vi "Search threshold value.vi"(0 "Delta Matrix":T2=[[-1.0, 0.0, 0.0, 0.0, 0.0, 0.0, 0.0, 0.0, 0.0], [0.0, -1.0, 0.0, 0.0, 0.0, 0.0, 0.0, 0.0, 0.0], [0.0, 0.0, 0.0, 0.0, 0.0, 0.0, 0.0, 0.0, 0.0], [0.0, 0.0, 0.0, 0.0, 0.0, 0.0, 0.0, 0.0, 0.0], [10.0, 0.0, 0.0, 0.0, 0.0, 0.0, 0.0, 0.0, 0.0], [10.0, 0.0, 0.0, 0.0, 0.0, 0.0, 0.0, 0.0, 0.0], [0.0, 10.0, 0.0, 0.0, 0.0, 0.0, 0.0, 0.0, 0.0]], 1 "Idx of Mod in Sp IDs":i32[](array[numeric])=[2, 8], 2 "CompID":string[](array[string]), 3 "CompSize":string[](array[string]), 5 "Equations":string[](array[string])=["kd*CI", "kd*GFP", "kd*LacI", "kd*TetR", "(ko__P1*ng__P1*Ko__P1*RNAP)/(1+Ko__P1*RNAP+(Kr__LacI_P1*LacI)^nc__LacI_P1)", "(ko__P2*ng__P2*Ko__P2*RNAP)/(1+Ko__P2*RNAP+(Kr__TetR_P2*TetR)^nc__TetR_P2)", "(ko__Promoter_GFP*ng__Promoter_GFP*Ko__Promoter_GFP*RNAP)/(1+Ko__Promoter_GFP*RNAP+(Kr__CI_Promoter_GFP*CI)^nc__CI_Promoter_GFP)"], 7 "Species Info":string[][](array[string])=[["CI", "", "0"], ["GFP", "", "0"], ["LacI", "", "0"], ["P1", "", "4"], ["P2", "", "2"], ["P3", "", "2"], ["P3_mRNA", "", "0"], ["Promoter_GFP", "", "2"], ["TetR", "", "0"]], 9 "Parameter info":string[][](array[string])=[["ko_r", "Reverse RNAP binding rate", "1", "", "", ""], ["nr", "Initial RNAP count", "30", "", "", ""], ["np", "Stoichiometry of production", "10", "", "", ""], ["kr_r", "Reverse repression binding rate", "1", "", "", ""], ["ka_f", "Forward activation binding rate", "0.0033", "", "", ""], ["kecdiff", "Extracellular diffusion rate", "1", "", "", ""], ["ko", "Open complex production rate", "0.05", "", "", ""], ["kmdiff_f", "Forward membrane diffusion rate", "1", "", "", ""], ["kecd", "Extracellular degradation rate", "0.005", "", "", ""], ["kc_r", "Reverse complex formation rate", "1", "", "", ""], ["kr_f", "Forward repression binding rate", "0.5", "", "", ""], ["ka_r", "Reverse activation binding rate", "1", "", "", ""], ["nc", "Stoichiometry of binding", "2", "", "", ""], ["kao_r", "Reverse activated RNAP binding rate", "1", "", "", ""], ["kd", "Degradation rate", "0.0075", "", "", ""], ["kb", "Basal production rate", "0.0001", "", "", ""], ["ng", "Initial promoter count", "2", "", "", ""], ["ka", "Activated production rate", "0.255", "", "", ""], ["kao_f", "Forward activated RNAP binding rate", "1", "", "", ""], ["kmdiff_r", "Reverse membrane diffusion rate", "0.01", "", "", ""], ["ko_f", "Forward RNAP binding rate", "0.033", "", "", ""], ["kc_f", "Forward complex formation rate", "0.05", "", "", ""], ["High", "", "60", "", "", ""], ["HighTime", "Reverse RNAP binding rate", "2000", "", "", ""], ["HighTime2", "Initial RNAP count", "4000", "", "", ""], ["", "", "", "ko_r", "Reverse RNAP binding rate", "1"], ["", "", "", "nr", "Initial RNAP count", "30"], ["", "", "", "np", "Stoichiometry of production", "10"], ["", "", "", "kr_r", "Reverse repression binding rate", "1"], ["", "", "", "ka_f", "Forward activation binding rate", "0.0033"], ["", "", "", "kecdiff", "Extracellular diffusion rate", "1"], ["", "", "", "ko", "Open complex production rate", "0.05"], ["", "", "", "kmdiff_f", "Forward membrane diffusion rate", "1"], ["", "", "", "kecd", "Extracellular degradation rate", "0.005"], ["", "", "", "kc_r", "Reverse complex formation rate", "1"], ["", "", "", "kr_f", "Forward repression binding rate", "0.5"], ["", "", "", "ka_r", "Reverse activation binding rate", "1"], ["", "", "", "nc", "Stoichiometry of binding", "2"], ["", "", "", "kao_r", "Reverse activated RNAP binding rate", "1"], ["", "", "", "kd", "Degradation rate", "0.0075"], ["", "", "", "kb", "Basal production rate", "0.0001"], ["", "", "", "ng", "Initial promoter count", "2"], ["", "", "", "ka", "Activated production rate", "0.255"], ["", "", "", "kao_f", "Forward activated RNAP binding rate", "1"], ["", "", "", "kmdiff_r", "Reverse membrane diffusion rate", "0.01"], ["", "", "", "ko_f", "Forward RNAP binding rate", "0.033"], ["", "", "", "kc_f", "Forward complex formation rate", "0.05"], ["", "", "", "High", "", "60"], ["", "", "", "HighTime", "Reverse RNAP binding rate", "2000"], ["", "", "", "HighTime2", "Initial RNAP count", "4000"]], 11 "Local Parameter Info":string[][](array[string])=[["kd", "0.0075", "0.0075", "0.0075"], ["kd", "0.0075", "0.0075", "0.0075"], ["kd", "0.0075", "0.0075", "0.0075"], ["kd", "0.0075", "0.0075", "0.0075"], ["RNAP", "30", "0.0075", "0.0075"], ["ng__P1", "4", "0.0075", "0.0075"], ["Ko__P1", "0.033", "0.0075", "0.0075"], ["ko__P1", "0.05", "0.0075", "0.0075"], ["nc__LacI_P1", "2", "0.0075", "0.0075"], ["Kr__LacI_P1", "0.5", "0.0075", "0.0075"], ["RNAP", "30", "0.0075", "0.0075"], ["ng__P2", "2", "0.0075", "0.0075"], ["Ko__P2", "0.033", "0.0075", "0.0075"], ["ko__P2", "0.05", "0.0075", "0.0075"], ["nc__TetR_P2", "2", "0.0075", "0.0075"], ["Kr__TetR_P2", "0.5", "0.0075", "0.0075"], ["RNAP", "30", "0.0075", "0.0075"], ["ng__Promoter_GFP", "2", "0.0075", "0.0075"], ["Ko__Promoter_GFP", "0.033", "0.0075", "0.0075"], ["ko__Promoter_GFP", "0.05", "0.0075", "0.0075"], ["nc__CI_Promoter_GFP", "2", "0.0075", "0.0075"], ["Kr__CI_Promoter_GFP", "0.5", "0.0075", "0.0075"], ["0.0075", "0.0075", "kd", "0.0075"], ["0.0075", "0.0075", "kd", "0.0075"], ["0.0075", "0.0075", "kd", "0.0075"], ["0.0075", "0.0075", "kd", "0.0075"], ["0.0075", "0.0075", "RNAP", "30"], ["0.0075", "0.0075", "ng__P1", "4"], ["0.0075", "0.0075", "Ko__P1", "0.033"], ["0.0075", "0.0075", "ko__P1", "0.05"], ["0.0075", "0.0075", "nc__LacI_P1", "2"], ["0.0075", "0.0075", "Kr__LacI_P1", "0.5"], ["0.0075", "0.0075", "RNAP", "30"], ["0.0075", "0.0075", "ng__P2", "2"], ["0.0075", "0.0075", "Ko__P2", "0.033"], ["0.0075", "0.0075", "ko__P2", "0.05"], ["0.0075", "0.0075", "nc__TetR_P2", "2"], ["0.0075", "0.0075", "Kr__TetR_P2", "0.5"], ["0.0075", "0.0075", "RNAP", "30"], ["0.0075", "0.0075", "ng__Promoter_GFP", "2"], ["0.0075", "0.0075", "Ko__Promoter_GFP", "0.033"], ["0.0075", "0.0075", "ko__Promoter_GFP", "0.05"], ["0.0075", "0.0075", "nc__CI_Promoter_GFP", "2"], ["0.0075", "0.0075", "Kr__CI_Promoter_GFP", "0.5"]], 12 "Inputs":T1={"Start at"=0.0, "Increment of"=5.0, "Stop at"=15.0, "No. of iterations"=10.0, "Assumed Time Delay"=800.0, "Th high"=0.0, "Verification RT"=1000.0, "Settling Time"=10, "Name of Output"="GFP", "Th Low"=90.0}, 13 "ModTimeSym":string) -> (4 "Estimated T-delay":i32, 6 "Th-High":dbl, 8 "ET-Delay-SD":dbl format="%0.2f", 10 "E-OC-Th-High":dbl format="%#_4g", 14 "E-OC-Th-Low":dbl, 15 "Th-Low":dbl)   [LabVIEW 2014]
doc: "This VI checks for the possible threshold value for two input genetic circuits. If any possible threshold value is detected, it triggers \"Verify threshold value by repeated iteration.vi\" to perform iterations and verify the level of consistency. \n\n\nLimitations:\n* Index of output protein is hard coded to GFP\n* Input combinations are hard coded for two input circuits\n*\n\nNote: \nLimitations:\n* Index of output protein is hard coded to GFP.\n* Input combinations are hard coded for two input circuits.\n\nDesigned by HB\nhaba@dtu.dk"
uses:
  <vilib>/Analysis/Matrix/Datatypes/RealMatrix.ctl
  Threshold Set.ctl
  ValSubsCtrl.ctl
  VerifyThreshInpCtrl.ctl
  Trigger Status Bar.vi
  <vilib>/Analysis/Matrix/Numeric/Conversions/Matrix To Array - RM.vi
  <vilib>/gmath/NI_Gmath.lvlib
  <vilib>/Analysis/Matrix/NI_Matrix.lvlib
panel:
  out "TIME IN MS":i32
  out "UD-OC-Th-Low":dbl
  out "OP Cons-Int":dbl
  in  "ThLow":bool
  out "Verification RT":dbl=1000.0
  out "Combinations":string[](array[string])
  out "UD-OC-Th-High":dbl
  out "output variable":u8
  out "Comb":string
  out "Init Sp State":i32[](array[numeric])
  out "Pos Thresh":dbl
  out "O/p cross":bool
  out "C-o/p":dbl
  out "Nxt Level":dbl
  out "Init OP Conc":dbl
  out "OP Data":dbl[](array[numeric])
  out "idx of OP":i32
  out "Level Run":i32
  out "Time Delay":dbl
  out "Levels":dbl format="%#_2g"
  out "Stop at":dbl
  out "Increment of":dbl
  out "Runs":dbl
  out "Start at":dbl
  out "Mod data":dbl[](array[numeric])
  out "Log Data matrix":dbl[][](array[numeric]) format="%0.3f"
  out "Sp Ids":string[](array[string])=["CI", "GFP", "LacI", "P1", "P2", "P3", "P3_mRNA", "Promoter_GFP", "TetR"]
  out "All Param Names":string[](array[string])
  out "All Param Values":string[](array[string])
  out "Nxt Sp State (N)":i32[](array[numeric])
  out "Nxt Sp State (S)":string[](array[string])
  out "Nxt T":dbl
  out "Sum of Propensities for U":dbl
  out "Reac to execute":dbl[](array[numeric])
  out "Output Equations":string[](array[string])
  out "Log Data":dbl[](array[numeric])
  out "Sum>a0*r2":bool
  out "Reac IDx":i32
  out "a0*r2":dbl
  out "r1":dbl
  out "a0":dbl
  out "Propensities":dbl[](array[numeric])
  out "L_cnt":i32
  out "T":dbl[](array[numeric])
  out "tau":dbl
  out "r2":dbl
  # "Inputs to \"iterative average calc July 20\"vi"
  # "Outputs from \"iterative average calc July 20\"vi"
  # "Delta Matrix"
  # "Start at"
  # "T-Delay"
  # "OP Consistency"
  # "Pos Thresh"
  # "Idx of Mod in Sp IDs"
  # "Runs"
  # "idx of OP"
  # "init Sp State"
  # "Equations"
  # "All Param Names"
  # "All Param Values"
  # "Sp IDs"
  # "Init OP Conc"
  # "Input concentration values"
  # "% Acceptance of consistency"
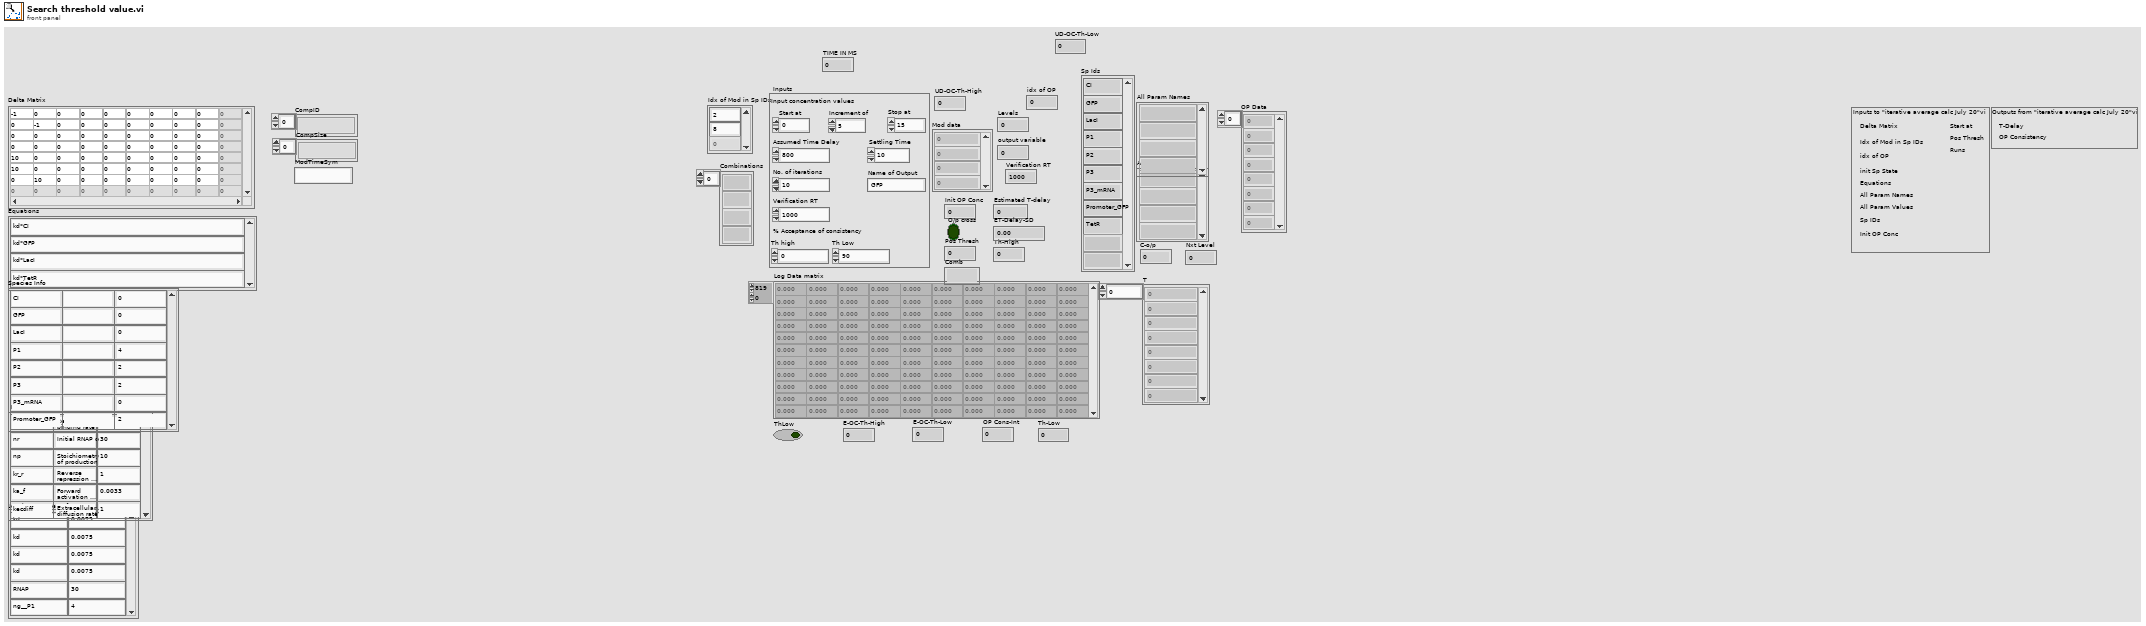
[diagram p1: front panel]
types:
  T1 = typedef "Threshold Set.ctl" = cluster{"Start at":dbl, "Increment of":dbl, "Stop at":dbl, "No. of iterations":dbl, "Assumed Time Delay":dbl, "Th high":dbl, "Verification RT":dbl, "Settling Time":i32, "Name of Output":string, "Th Low":dbl}
  T2 = typedef "NI_Matrix.lvlib/RealMatrix.ctl" = dbl[][]
  T3 = typedef "ValSubsCtrl.ctl" = cluster{"All Param Names":string[], "All Param Values":string[], "Sp IDs":string[], "Sp States":string[], "Input Equations":string[], "CompID":string[], "CompSize":string[], "T-Sym":string, "T":dbl}
  T4 = typedef "VerifyThreshInpCtrl.ctl" = cluster{"Delta Matrix ":T2, "Idx of Mod in Sp IDs ":i32[], "idx of OP ":i32, "Init Sp State ":i32[], "Equations ":string[], "All Param Names ":string[], "All Param Values ":string[], "Sp Ids ":string[], "Start at ":dbl, "Pos Thresh ":dbl, "Runs ":dbl, "Init OP Conc ":dbl, "Comb ":string, "Verification RT ":dbl, "CompID":string[], "CompSize":string[], "ModTimeSym":string, "Settling Time":i32}
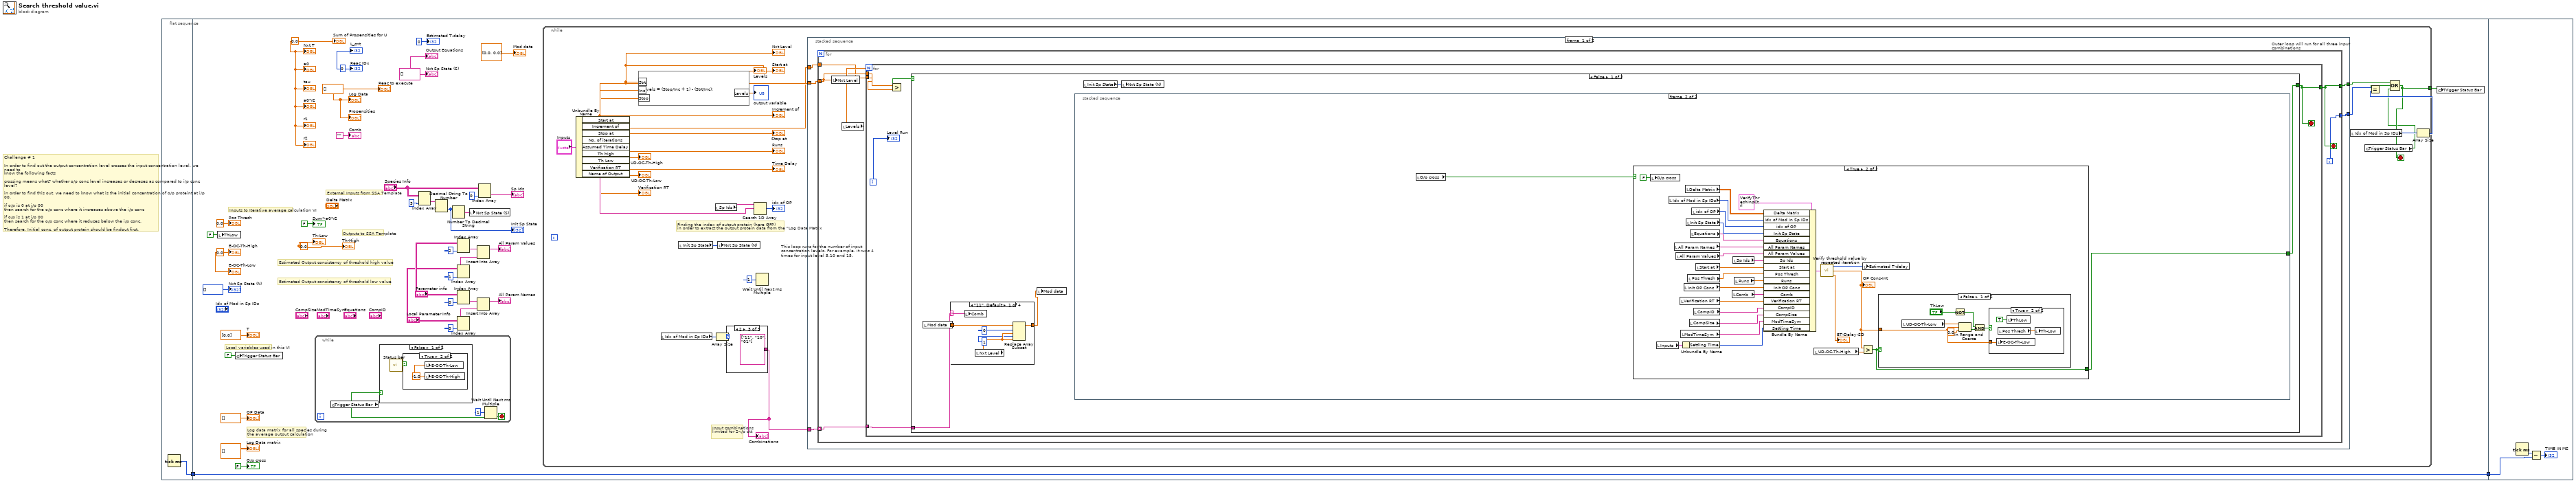
[diagram p0: block diagram]
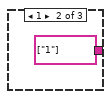
[diagram p5: hidden frame]
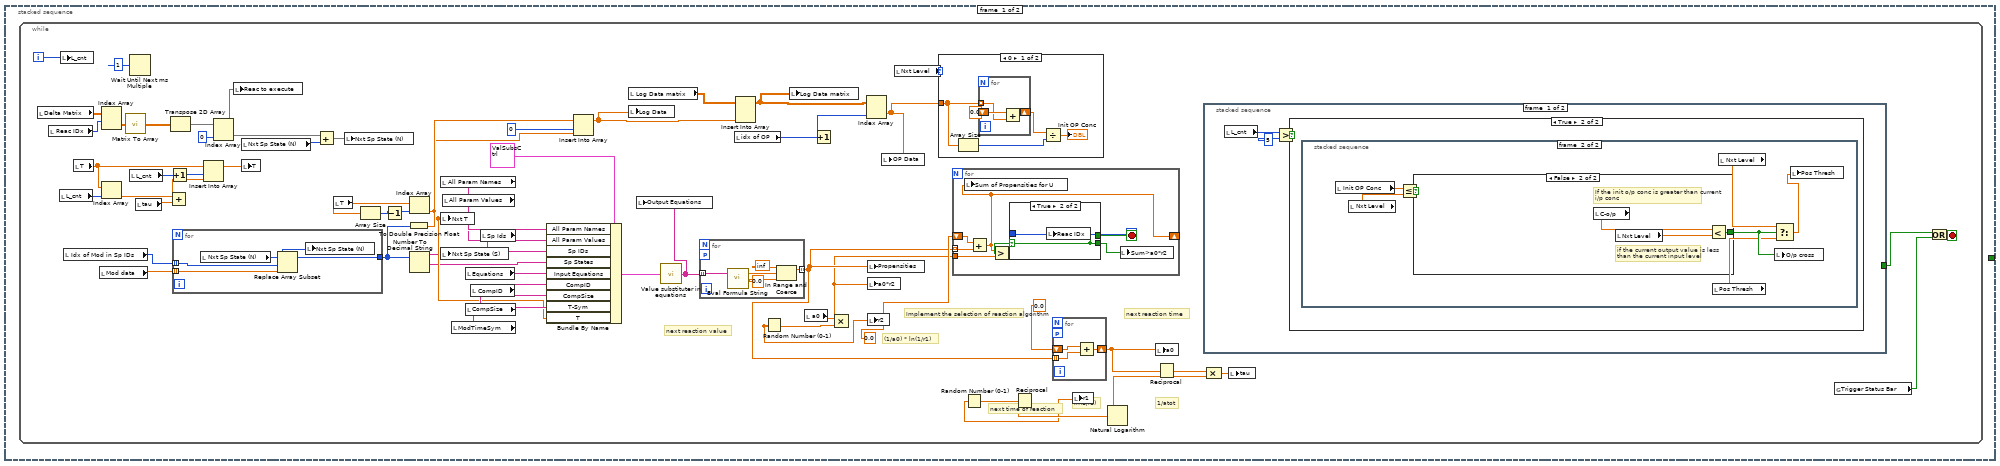
[diagram p6: hidden frame]
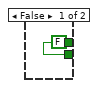
[diagram p8: hidden frame]
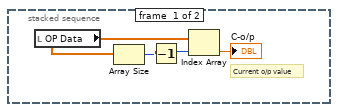
[diagram p10: hidden frame]
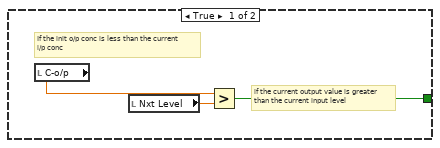
[diagram p11: hidden frame]
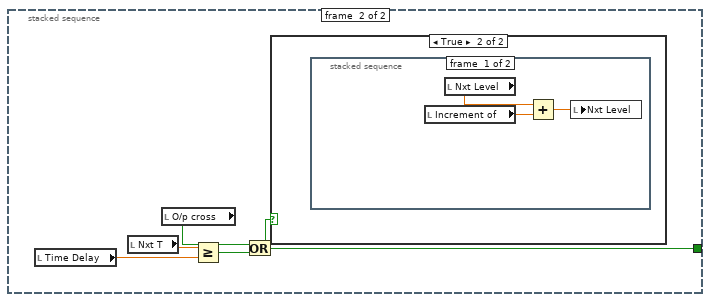
[diagram p12: hidden frame]
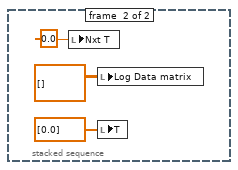
[diagram p14: hidden frame]
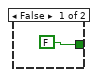
[diagram p15: hidden frame]
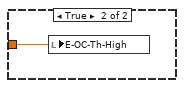
[diagram p17: hidden frame]
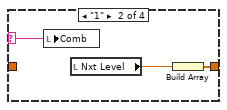
[diagram p18: hidden frame]
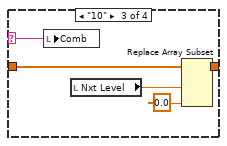
[diagram p19: hidden frame]
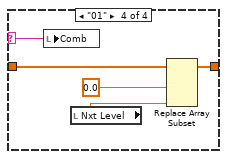
[diagram p20: hidden frame]
diagram:
  # "Challenge # 1\n\nIn order to find out the output concentration level crosses the input concentration level, we need to \nknow the following facts\n\ncrossing means what? whether o/p conc level increases or decreses as compared to i/p conc level?\n\nin order to find this out, we need to know what is the initial concentration of o/p proteint at i/p 00.\n\nif o/p is 0 at i/p 00\nthen search for the o/p conc where it increases above the i/p conc\n\nif o/p is 1 at i/p 00\nthen search for the o/p conc where it reduces below the i/p conc.\n\nTherefore, Initial conc. of output protein should be findout first."
  n1 = flat-sequence {
    tunnel: [w3] -> w1
    tunnel: [w4] -> w2
    tunnel: w1 -> [w4]
    tunnel: w2 -> [w281]
    frame #0 {
      n2 = Tick Count (ms)() -> (millisecond timer value=w3:u32)
    }
    frame #1 {
      w6 = 0.0 ("OP Consistency (%)")
      w5 = 0.0 ("Threshold Value")
      w17 = dbl[] [] ("Reac to execute")
      w28 = 0.0 ("a0")
      w29 = 0 ("L_cnt")
      w30 = string[] [] ("Nxt Sp State (S)")
      # "Estimated Output consistency of threshold low value"
      # "Estimated Output consistency of threshold high value"
      # "Local variables used in this VI"
      # "Outputs to SSA Template"
      # "Log data matrix for all species during \nthe average output calculation"
      # "Inputs to Iterative average calculation VI"
      # "External Inputs from SSA Template"
      n3 = local write "ThLow"(FALSE ("ThLow")) -> ()
      n4 = global write "Trigger Status Bar.vi" "Trigger Status Bar"(FALSE ("Trigger Status Bar")) -> ()
      n5 = while {
        stop <- w44 stop-if-true
        n6 = global read "Trigger Status Bar.vi" "Trigger Status Bar"() -> (w44:bool)
        n7 = case shown="False" w44 {
          frame False {
            n8 = call "Status bar.vi"() -> ("Cancel Button 2"=w45:bool)  [unwired: 11 in]
            n9 = case shown="True" w45 {
              frame False {
              }
              frame True {
                w46 = -1.0 ("OP Consistency (%)")
                n10 = local write "E-OC-Th-Low"(w46) -> ()
                n11 = local write "E-OC-Th-High"(w46) -> ()
              }
            }
          }
          frame True {
          }
        }
        n12 = Wait Until Next ms Multiple(millisecond multiple=u32 1) -> ()  [unwired: 1 out]
      }
      n13 = Index Array(array="Species Info", index (col)=3 ("disabled index (col)")) -> (element=w24:string[])  [unwired: 1 in]
      n14 = Decimal String To Number(string=w24) -> (number=w21:i32[])  [unwired: 2 in, 1 out]
      "Init Sp State" <- w21
      n15 = Number To Decimal String(number=w21) -> (decimal integer string=w20:string[])  [unwired: 1 in]
      n16 = Index Array(array="Parameter info", index (col)=2 ("disabled index (col)")) -> (element=w36:string[])  [unwired: 1 in]
      n17 = Index Array(array="Local Parameter Info", index (col)=1 ("disabled index (col)")) -> (element=w35:string[])  [unwired: 1 in]
      n18 = Index Array(array="Parameter info", index (col)=0 ("disabled index (col)")) -> (element=w38:string[])  [unwired: 1 in]
      n19 = Index Array(array="Local Parameter Info", index (col)=0 ("disabled index (col)")) -> (element=w37:string[])  [unwired: 1 in]
      n20 = local write "Nxt Sp State (S)"(w20) -> ()
      n21 = Insert Into Array(array=w36, new element=w35) -> (→"All Param Values":string[])  [unwired: 1 in]
      n22 = Insert Into Array(array=w38, new element=w37) -> (→"All Param Names":string[])  [unwired: 1 in]
      n23 = Index Array(array="Species Info", index (col)=0 ("disabled index (col)")) -> (element=→"Sp Ids":string[])  [unwired: 1 in]
      n24 = while {
        tunnel: [w65] -> w8
        stop <- w65 stop-if-true
        # "Input combinations\nlimited for 2-i/p ckt"
        # "Finding the index of output protein (here GFP)\nin order to extract the output protein data from the \"Log Data Matrix"
        n25 = Unbundle By Name("Inputs") -> ("Start at"=w49:dbl, "Increment of"=w52:dbl, "Stop at"=w47:dbl, "No. of iterations"=→"Runs":dbl, "Assumed Time Delay"=→"Time Delay":dbl, "Th high"=→"UD-OC-Th-High":dbl, "Th Low"=→"UD-OC-Th-Low":dbl, "Verification RT"=→"Verification RT":dbl, "Name of Output"=w59:string)
        "Start at" <- w49
        "Increment of" <- w52
        "Stop at" <- w47
        "Nxt Level" <- w49
        n26 = formula code="Levels = (Stop/Inc + 1) - (Strt/Inc);"("Strt"=w49, "Inc"=w52, "Stop"=w47) -> ("Levels"=→"Levels" →"output variable":dbl)
        n27 = local read "Idx of Mod in Sp IDs"() -> (w62:i32[])
        n28 = local read "Init Sp State"() -> (w61:i32[])
        n29 = local read "Sp Ids"() -> (w57:string[])
        n30 = Array Size(array=w62) -> (size(s)=w63:i32)
        n31 = local write "Nxt Sp State (N)"(w61) -> ()
        n32 = case shown="2" w63 {
          tunnel: [_ string[] ["1"] string[] ["11", "10", "01"]] -> w48
          frame 0, Default {
          }
          frame 1 {
          }
          frame 2 {
          }
        }
        "Combinations" <- w48
        n33 = Search 1D Array(1D array=w57, element=w59) -> (index of element=→"idx of OP":i32)  [unwired: 1 in]
        n34 = Wait Until Next ms Multiple(millisecond multiple=u32 1) -> ()  [unwired: 1 out]
        n35 = stacked-sequence {
          tunnel: [w78 _] -> w70
          tunnel: [w77 _] -> w71
          tunnel: w49 -> [w76 _]
          tunnel: w48 -> [w75 _]
          tunnel: w47 -> [w74 _]
          frame #0 {
            n36 = for "Outer loop will run for all three input combinations" {
              tunnel: w75 -> [w84] mode=indexing
              tunnel: w76 -> [w80]
              tunnel: [w82] -> w78
              tunnel: [w81] -> w77
              tunnel: w74 -> [w79]
              i -> [w81]
              stop <- w82 stop-if-true
              n37 = local write "Nxt Level"(w80) -> ()
              n38 = local read "Levels"() -> (w83:dbl)
              n39 = for "This loop runs for the number of input concentration levels. For example, it runs 4 times for input level 5,10 and 15." {
                N: w83 -> [_]
                tunnel: w84 -> [w90]
                tunnel: [w87] -> w82
                tunnel: w80 -> [w86]
                tunnel: w79 -> [w85]
                i -> [w89]
                stop <- w87 stop-if-true
                n40 = Greater?(x=w86, y=w85) -> (0:w88:bool)
                n41 = case shown="False" w88 {
                  selector: w88 -> [_ w279]
                  tunnel: w90 -> [w95 _]
                  tunnel: [w94 w279] -> w87
                  frame False {
                    n42 = local read "Mod data"() -> (w92:dbl[])
                    n43 = case shown="\"11\", Default" w95 {
                      selector: w95 -> [w260 w266 w269 w274]
                      tunnel: w92 -> [w265 _ w273 w278]
                      tunnel: [w264 w267 w272 w277] -> w93
                      frame "11", Default {
                        n44 = local write "Comb"(w260) -> ()
                        n45 = local read "Nxt Level"() -> (w263:dbl)
                        n46 = Replace Array Subset(array=w265, new element #1=w263, index #1=0 ("index"), new element #2=w263, index #2=1 ("index")) -> (w264:dbl[])
                      }
                      frame "1" {
                        n47 = local write "Comb"(w266) -> ()
                        n48 = local read "Nxt Level"() -> (w268:dbl)
                        n49 = Build Array(w268) -> (w267:dbl[])
                      }
                      frame "10" {
                        n50 = local write "Comb"(w269) -> ()
                        n51 = local read "Nxt Level"() -> (w270:dbl)
                        n52 = Replace Array Subset(array=w273, new element #1=w270, new element #2=0.0 ("new element/subarray")) -> (w272:dbl[])  [unwired: 2 in]
                      }
                      frame "01" {
                        n53 = local write "Comb"(w274) -> ()
                        n54 = local read "Nxt Level"() -> (w275:dbl)
                        n55 = Replace Array Subset(array=w278, new element #1=0.0 ("new element/subarray"), new element #2=w275) -> (w277:dbl[])  [unwired: 2 in]
                      }
                    }
                    n56 = local write "Mod data"(w93) -> ()
                    n57 = stacked-sequence {
                      tunnel: [_ w219] -> w94
                      frame #0 {
                        n58 = while {
                          i -> [w156]
                          stop <- w153 stop-if-true
                          # "Implement the selection of reaction algorithm"
                          # "(1/a0) * ln(1/r1)"
                          # "1/atot"
                          # "ln(1/r1)"
                          # "next reaction time"
                          # "next time of reaction"
                          # "next reaction value"
                          n59 = local read "Delta Matrix"() -> (w109:T2)
                          n60 = local read "Reac IDx"() -> (w108:i32)
                          n61 = local read "L_cnt"() -> (w124:i32)
                          n62 = local write "L_cnt"(w156) -> ()
                          n63 = local read "Idx of Mod in Sp IDs"() -> (w150:i32[])
                          n64 = local read "T"() -> (w113:dbl[])
                          n65 = local read "Mod data"() -> (w151:dbl[])
                          n66 = Index Array(array=w109, index (row)=w108) -> (element=w107:T2)  [unwired: 1 in]
                          n67 = Index Array(array=w113, index=w124) -> (element=w122:dbl)
                          n68 = call-poly <vilib>:"Matrix To Array.vi"("Real Matrix"=w107) -> ("Real 2D Array"=w106:dbl[][])
                          n69 = local read "L_cnt"() -> (w120:i32)
                          n70 = Wait Until Next ms Multiple(millisecond multiple=u32 1) -> ()  [unwired: 1 out]
                          n71 = local read "tau"() -> (w123:dbl)
                          n72 = Add(x=w122, y=w123) -> (x+y=w119:dbl)
                          n73 = Increment(x=w120) -> (x+1=w121:i32)
                          n74 = Transpose 2D Array(2D array=w106) -> (transposed array=w105:dbl[][])
                          n75 = for {
                            tunnel: w150 -> [w186] mode=indexing
                            tunnel: w151 -> [w185] mode=indexing
                            tunnel: [w184] -> w143
                            n76 = local read "Nxt Sp State (N)"() -> (w187:i32[])
                            n77 = Replace Array Subset(array=w187, new element=w185, index=w186) -> (w184:i32[])
                            n78 = local write "Nxt Sp State (N)"(w184) -> ()
                          }
                          n79 = Insert Into Array(array=w113, index=w121, new element=w119) -> (w118:dbl[])
                          n80 = Index Array(array=w105, index (col)=0 ("disabled index (col)")) -> (element=w101:dbl[])  [unwired: 1 in]
                          n81 = local write "Reac to execute"(w101) -> ()
                          n82 = local read "Nxt Sp State (N)"() -> (w103:i32[])
                          n83 = local write "T"(w118) -> ()
                          n84 = Add(x=w101, y=w103) -> (x+y=w102:dbl[])
                          n85 = local read "T"() -> (w149:dbl[])
                          n86 = local write "Nxt Sp State (N)"(w102) -> ()
                          n87 = Array Size(array=w149) -> (size(s)=w148:i32)
                          n88 = Decrement(x=w148) -> (x-1=w147:i32)
                          n89 = Index Array(array=w149, index=w147) -> (element=w130:dbl)
                          n90 = To Double Precision Float(number=w143) -> (double precision float=w145:dbl[])
                          n91 = Number To Decimal String(number=w143) -> (decimal integer string=w129:string[])  [unwired: 1 in]
                          n92 = local read "All Param Names"() -> (w137:string[])
                          n93 = local write "Nxt T"(w130) -> ()
                          n94 = local write "Nxt Sp State (S)"(w129) -> ()
                          n95 = local read "All Param Values"() -> (w136:string[])
                          n96 = local read "ModTimeSym"() -> (w141:string)
                          n97 = local read "Equations"() -> (w138:string[])
                          n98 = local read "CompSize"() -> (w140:string[])
                          n99 = local read "CompID"() -> (w139:string[])
                          n100 = local read "Sp Ids"() -> (w135:string[])
                          n101 = Bundle By Name(cluster=T3 {"All Param Names"=["k1"], "All Param Values"=["1.5"], "Sp IDs"=["S1", "S2", "S3"], "Sp States"=["0.000000", "0.000000", "0.000000"], "Input Equations"=["C*k1*S1", "1.5*exp(time)^(-1)"], "CompID"=["C"], "CompSize"=["3.0"], "T-Sym"="time", "T"=0.0} ("Cluster"), "All Param Names"=w137, "All Param Values"=w136, "Sp IDs"=w135, "Sp States"=w129, "Input Equations"=w138, "CompID"=w139, "CompSize"=w140, "T-Sym"=w141, "T"=w130) -> (w134:T3)
                          n102 = Insert Into Array(array=w145, index=0, new element=w130) -> (w142:dbl[])
                          n103 = local read "Log Data matrix"() -> (w144:dbl[][])
                          n104 = local write "Log Data"(w142) -> ()
                          n105 = call "Value substituter in equations.vi"("Cluster"=w134) -> ("Output Equations"=w131:string[])
                          n106 = local write "Output Equations"(w131) -> ()
                          n107 = for {
                            tunnel: w131 -> [w183] mode=indexing
                            tunnel: [w179] -> w111 mode=indexing
                            workers-P: _ -> [_]
                            n108 = call <vilib>:"Eval Formula String.vi"("formula"=w183) -> ("y value"=w180:dbl)  [unwired: 1 in, 1 out]
                            n109 = In Range and Coerce(upper limit=inf, x=w180, lower limit=0.0) -> (coerced(x)=w179:dbl)  [unwired: 1 out]
                          }
                          n110 = local read "idx of OP"() -> (w97:i32)
                          n111 = Insert Into Array(array=w144, new element=w142) -> (w96:dbl[][])  [unwired: 2 in]
                          n112 = Random Number (0-1)() -> (number: 0 to 1=w114:dbl)
                          n113 = local write "Log Data matrix"(w96) -> ()
                          n114 = local read "a0"() -> (w117:dbl)
                          n115 = Increment(x=w97) -> (x+1=w98:i32)
                          n116 = Multiply(x=w117, y=w114) -> (x*y=w110:dbl)
                          n117 = Index Array(array=w96, index (col)=w98) -> (element=w100:dbl[])  [unwired: 1 in]
                          n118 = local write "Propensities"(w111) -> ()
                          n119 = local write "a0*r2"(w110) -> ()
                          n120 = local write "r2"(w114) -> ()
                          n121 = local write "OP Data"(w100) -> ()
                          n122 = local read "Nxt Level"() -> (w99:dbl)
                          n123 = case shown="0" w99 {
                            tunnel: w100 -> [w159 _]
                            frame 0 {
                              n124 = Array Size(array=w159) -> (size(s)=w158:i32)
                              n125 = for {
                                tunnel: w159 -> [w163] mode=indexing
                                shift-right: [w162] -> w160
                                shift-left: 0.0 -> [w164]
                                n126 = Add(x=w164, y=w163) -> (x+y=w162:dbl)
                              }
                              n127 = Divide(x=w160, y=w158) -> (x/y=→"Init OP Conc":dbl)
                            }
                            frame 1.., Default {
                            }
                          }
                          n128 = for {
                            tunnel: w111 -> [w169] mode=indexing
                            shift-right: [w168] -> _
                            shift-left: 0.0 -> [w172]
                            tunnel: w110 -> [w165]
                            i -> [w166]
                            stop <- w170 stop-if-true
                            n129 = Add(x=w172, y=w169) -> (x+y=w168:dbl)
                            n130 = local write "Sum of Propensities for U"(w168) -> ()
                            n131 = Greater?(x=w168, y=w165) -> (0:w171:bool)
                            n132 = case shown="True" w171 {
                              selector: w171 -> [_ w175]
                              tunnel: [w173 w175] -> w170
                              tunnel: [w173 w175] -> w167
                              tunnel: w166 -> [_ w174]
                              frame False {
                                w173 = FALSE
                              }
                              frame True {
                                n133 = local write "Reac IDx"(w174) -> ()
                              }
                            }
                            n134 = local write "Sum>a0*r2"(w167) -> ()
                          }
                          n135 = Random Number (0-1)() -> (number: 0 to 1=w115:dbl)
                          n136 = Reciprocal(x=w115) -> (1/x=w125:dbl)
                          n137 = for {
                            tunnel: w111 -> [w178] mode=indexing
                            shift-right: [w177] -> w116
                            shift-left: 0.0 -> [w176]
                            workers-P: _ -> [_]
                            n138 = Add(x=w176, y=w178) -> (x+y=w177:dbl)
                          }
                          n139 = local write "r1"(w115) -> ()
                          n140 = Natural Logarithm(1:w125) -> (0:w127:dbl)
                          n141 = local write "a0"(w116) -> ()
                          n142 = Reciprocal(x=w116) -> (1/x=w126:dbl)
                          n143 = stacked-sequence {
                            tunnel: [_ w208] -> w154
                            frame #0 {
                              n144 = local read "L_cnt"() -> (w189:i32)
                              n145 = Greater?(x=w189, y=5) -> (0:w190:bool)
                              n146 = case shown="True" w190 {
                                frame False {
                                }
                                frame True {
                                n147 = stacked-sequence {
                                frame #0 {
                                # "Current o/p value"
                                n148 = local read "OP Data"() -> (w192:dbl[])
                                n149 = Array Size(array=w192) -> (size(s)=w193:i32)
                                n150 = Decrement(x=w193) -> (x-1=w194:i32)
                                n151 = Index Array(array=w192, index=w194) -> (element=→"C-o/p":dbl)
                                }
                                frame #1 {
                                n152 = local read "Init OP Conc"() -> (w201:dbl)
                                n153 = local read "Nxt Level"() -> (w200:dbl)
                                n154 = Less Or Equal?(x=w201, y=w200) -> (x <= y?=w199:bool)
                                n155 = case shown="False" w199 {
                                tunnel: [w202 w205] -> w198
                                frame True {
                                # "if the current output value is greater\nthan the current input level"
                                # "If the init o/p conc is less than the current \ni/p conc"
                                n156 = local read "C-o/p"() -> (w204:dbl)
                                n157 = local read "Nxt Level"() -> (w203:dbl)
                                n158 = Greater?(x=w204, y=w203) -> (0:w202:bool)
                                }
                                frame False {
                                # "if the current output value is less\nthan the current input level"
                                # "If the init o/p conc is greater than current \ni/p conc"
                                n159 = local read "C-o/p"() -> (w207:dbl)
                                n160 = local read "Nxt Level"() -> (w206:dbl)
                                n161 = Less?(x=w207, y=w206) -> (x < y?=w205:bool)
                                }
                                }
                                n162 = local read "Pos Thresh"() -> (w195:dbl)
                                n163 = local read "Nxt Level"() -> (w197:dbl)
                                n164 = Select(t=w197, s=w198, f=w195) -> (s? t:f=w196:dbl)
                                n165 = local write "O/p cross"(w198) -> ()
                                n166 = local write "Pos Thresh"(w196) -> ()
                                }
                                }
                                }
                              }
                            }
                            frame #1 {
                              n167 = local read "Time Delay"() -> (w211:dbl)
                              n168 = local read "Nxt T"() -> (w212:dbl)
                              n169 = local read "O/p cross"() -> (w209:bool)
                              n170 = Greater Or Equal?(x=w212, y=w211) -> (x >= y?=w210:bool)
                              n171 = Or(x=w209, y=w210) -> (x .or. y?=w208:bool)
                              n172 = case shown="True" w208 {
                                frame False {
                                }
                                frame True {
                                n173 = stacked-sequence {
                                frame #0 {
                                n174 = local read "Increment of"() -> (w214:dbl)
                                n175 = local read "Nxt Level"() -> (w213:dbl)
                                n176 = Add(x=w213, y=w214) -> (x+y=w215:dbl)
                                n177 = local write "Nxt Level"(w215) -> ()
                                }
                                frame #1 {
                                n178 = local write "Nxt T"(0.0 ("Nxt T")) -> ()
                                n179 = local write "Log Data matrix"(dbl[][] [] ("Log Data matrix")) -> ()
                                n180 = local write "T"(dbl[] [0.0] ("T")) -> ()
                                }
                                }
                                }
                              }
                            }
                          }
                          n181 = Compound Arithmetic op=MULTIPLY(w126, w127) -> (w128:dbl)
                          n182 = local write "tau"(w128) -> ()
                          n183 = global read "Trigger Status Bar.vi" "Trigger Status Bar"() -> (w152:bool)
                          n184 = Or(x=w154, y=w152) -> (x .or. y?=w153:bool)
                        }
                      }
                      frame #1 {
                        n185 = local read "O/p cross"() -> (w220:bool)
                        n186 = case shown="True" w220 {
                          tunnel: [FALSE w248] -> w219
                          frame False {
                          }
                          frame True {
                            n187 = local write "O/p cross"(FALSE ("O/p cross")) -> ()
                            n188 = local read "Inputs"() -> (w223:T1)
                            n189 = local read "Idx of Mod in Sp IDs"() -> (w240:i32[])
                            n190 = local read "All Param Names"() -> (w236:string[])
                            n191 = local read "All Param Values"() -> (w235:string[])
                            n192 = local read "Verification RT"() -> (w228:dbl)
                            n193 = local read "ModTimeSym"() -> (w225:string)
                            n194 = Unbundle By Name(w223) -> ("Settling Time"=w222:i32)
                            n195 = local read "Init OP Conc"() -> (w230:dbl)
                            n196 = local read "Delta Matrix"() -> (w241:T2)
                            n197 = local read "Init Sp State"() -> (w238:i32[])
                            n198 = local read "Pos Thresh"() -> (w232:dbl)
                            n199 = local read "CompSize"() -> (w226:string[])
                            n200 = local read "Equations"() -> (w237:string[])
                            n201 = local read "idx of OP"() -> (w239:i32)
                            n202 = local read "CompID"() -> (w227:string[])
                            n203 = local read "Start at"() -> (w233:dbl)
                            n204 = local read "Comb"() -> (w229:string)
                            n205 = local read "Sp Ids"() -> (w234:string[])
                            n206 = local read "Runs"() -> (w231:dbl)
                            n207 = Bundle By Name(cluster=T4 {"Delta Matrix "=[[-1.0, 0.0, 0.0, 0.0, 0.0, 0.0, 0.0, 0.0, 0.0], [0.0, -1.0, 0.0, 0.0, 0.0, 0.0, 0.0, 0.0, 0.0], [0.0, 0.0, 0.0, 0.0, 0.0, 0.0, 0.0, 0.0, 0.0], [0.0, 0.0, 0.0, 0.0, 0.0, 0.0, 0.0, 0.0, 0.0], [10.0, 0.0, 0.0, 0.0, 0.0, 0.0, 0.0, 0.0, 0.0], [10.0, 0.0, 0.0, 0.0, 0.0, 0.0, 0.0, 0.0, 0.0], [0.0, 10.0, 0.0, 0.0, 0.0, 0.0, 0.0, 0.0, 0.0]], "Idx of Mod in Sp IDs "=[2, 8], "idx of OP "=0, "Init Sp State "=[], "Equations "=["kd*CI", "kd*GFP", "kd*LacI", "kd*TetR", "(ko__P1*ng__P1*Ko__P1*RNAP)/(1+Ko__P1*RNAP+(Kr__LacI_P1*LacI)^nc__LacI_P1)", "(ko__P2*ng__P2*Ko__P2*RNAP)/(1+Ko__P2*RNAP+(Kr__TetR_P2*TetR)^nc__TetR_P2)", "(ko__Promoter_GFP*ng__Promoter_GFP*Ko__Promoter_GFP*RNAP)/(1+Ko__Promoter_GFP*RNAP+(Kr__CI_Promoter_GFP*CI)^nc__CI_Promoter_GFP)"], "All Param Names "=[], "All Param Values "=[], "Sp Ids "=["CI", "GFP", "LacI", "P1", "P2", "P3", "P3_mRNA", "Promoter_GFP", "TetR"], "Start at "=0.0, "Pos Thresh "=10.0, "Runs "=0.0, "Init OP Conc "=0.0, "Comb "="", "Verification RT "=0.0, "CompID"=["C"], "CompSize"=["1.0"], "ModTimeSym"="", "Settling Time"=10} ("Cluster"), "Delta Matrix"=w241, "Idx of Mod in Sp IDs"=w240, "idx of OP"=w239, "Init Sp State"=w238, "Equations"=w237, "All Param Names"=w236, "All Param Values"=w235, "Sp Ids"=w234, "Start at"=w233, "Pos Thresh"=w232, "Runs"=w231, "Init OP Conc"=w230, "Comb"=w229, "Verification RT"=w228, "CompID"=w227, "CompSize"=w226, "ModTimeSym"=w225, "Settling Time"=w222) -> (w242:T4)
                            n208 = local read "UD-OC-Th-High"() -> (w244:dbl)
                            n209 = call "Verify threshold value by repeated iteration.vi"("Cluster"=w242) -> ("T-Delay-SD"=→"ET-Delay-SD":dbl, "OP Consistency"=w245:dbl, "T-delay.av"=w246:i32)  [unwired: 2 in]
                            "OP Cons-Int" <- w245
                            n210 = Greater?(x=w245, y=w244) -> (0:w248:bool)
                            n211 = local write "Estimated T-delay"(w246) -> ()
                            n212 = case shown="False" w248 {
                              tunnel: w245 -> [w250 w259]
                              frame False {
                                n213 = local read "UD-OC-Th-Low"() -> (w249:dbl)
                                n214 = Not(x="ThLow") -> (.not. x?=w254:bool)
                                n215 = In Range and Coerce(upper limit=w249, x=w250, lower limit=0.0 ("OP Consistency (%)")) -> (In Range?=w251:bool)  [unwired: 1 out]
                                n216 = And(x=w254, y=w251) -> (x .and. y?=w255:bool)
                                n217 = case shown="True" w255 {
                                tunnel: w250 -> [_ w256]
                                frame False {
                                }
                                frame True {
                                n218 = local write "E-OC-Th-Low"(w256) -> ()
                                n219 = local read "Pos Thresh"() -> (w257:dbl)
                                n220 = local write "ThLow"(TRUE ("ThLow")) -> ()
                                n221 = local write "Th-Low"(w257) -> ()
                                }
                                }
                              }
                              frame True {
                                n222 = local write "E-OC-Th-High"(w259) -> ()
                              }
                            }
                          }
                        }
                      }
                    }
                    n223 = local read "Init Sp State"() -> (w91:i32[])
                    n224 = local write "Nxt Sp State (N)"(w91) -> ()
                  }
                  frame True {
                  }
                }
                "Level Run" <- w89
              }
            }
          }
          frame #1 {
            n225 = local read "Pos Thresh"() -> (w280:dbl)
            n226 = local write "Th-High"(w280) -> ()
          }
        }
        n227 = local read "Idx of Mod in Sp IDs"() -> (w67:i32[])
        n228 = global read "Trigger Status Bar.vi" "Trigger Status Bar"() -> (w64:bool)
        n229 = Array Size(array=w67) -> (size(s)=w66:i32)
        n230 = Equal?(x=w71, y=w66) -> (x = y?=w69:bool)
        n231 = Compound Arithmetic op=OR(w70, w69, w64) -> (w65:bool)
      }
      n232 = global write "Trigger Status Bar.vi" "Trigger Status Bar"(w8) -> ()
      "r2" <- w28
      "tau" <- w28
      "T" <- dbl[] [0.0] ("T")
      "L_cnt" <- w29
      "Propensities" <- w17
      "a0" <- w28
      "r1" <- w28
      "a0*r2" <- w28
      "Reac IDx" <- w29
      "Sum>a0*r2" <- FALSE ("Sum>a0*r2")
      "Log Data" <- w17
      "Output Equations" <- w30
      "Reac to execute" <- w17
      "Sum of Propensities for U" <- w28
      "Nxt T" <- w28
      "Nxt Sp State (S)" <- w30
      "Nxt Sp State (N)" <- i32[] [] ("Nxt Sp State (N)")
      "Log Data matrix" <- dbl[][] [] ("Log Data matrix")
      "Mod data" <- dbl[] [0.0, 0.0] ("Mod data")
      "O/p cross" <- FALSE ("O/p cross")
      "OP Data" <- dbl[] [] ("OP Data")
      "Pos Thresh" <- 0.0 ("Pos Thresh")
      "Estimated T-delay" <- 0 ("T-delay")
      "Th-High" <- w5
      "E-OC-Th-High" <- w6
      "Comb" <- ""
      "Th-Low" <- w5
      "E-OC-Th-Low" <- w6
    }
    frame #2 {
      n233 = Tick Count (ms)() -> (millisecond timer value=w283:u32)
      n234 = Subtract(x=w283, y=w281) -> (x-y=→"TIME IN MS":u32)
    }
  }
